vi "VSI Slave Read Bytes.vi"(8 "error in (no error)":errorcluster, 9 "WaitTime":i32, 10 "DevIndex":i32, 11 "DevType":i32) -> (0 "error out":errorcluster, 1 "function return":i32, 2 "pBytesNum":i32, 3 "pReadData":string)   [LabVIEW 2012, in "ControlSPI.lvlib"]
doc: "int WINAPI VSI_SlaveReadBytes(int DevType,int DevIndex,unsigned char *pReadData,int *pBytesNum,int WaitTime);"
uses:
  ControlSPI.lvlib
  Ginkgo_Driver.dll
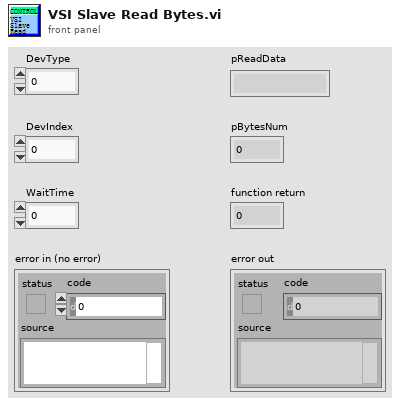
[diagram p1: front panel]
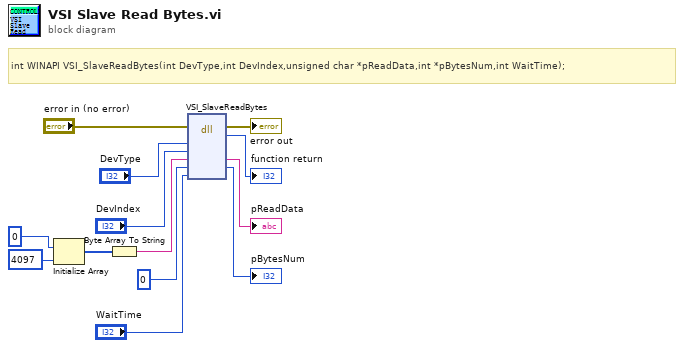
[diagram p0: block diagram]
diagram:
  # "int WINAPI VSI_SlaveReadBytes(int DevType,int DevIndex,unsigned char *pReadData,int *pBytesNum,int WaitTime);"
  n1 = Initialize Array(u8 0 ("element"), 4097 ("dimension size")) -> (w10:u8[])
  n2 = Byte Array To String(unsigned byte array=w10) -> (string=w9:string)
  n3 = dll-call lib="E:/Project/vt_ginkgo/truck/Ginkgo Driver/vs2010/Ginkgo_USB-I2C_API_v2.0.3.0/lib/labview_32bit/ControlSPI/Ginkgo_Driver.*" fn="VSI_SlaveReadBytes"(error in="error in (no error)", "DevType"="DevType", "DevIndex"="DevIndex", "pReadData"=w9, "pBytesNum"=0, "WaitTime"="WaitTime") -> (error out=→"error out":errorcluster, →"function return":i32, "pReadData"=→"pReadData":string, "pBytesNum"=→"pBytesNum":i32)  [unwired: 5 in, 1 out]
